vi "DEMO.vi"() -> ()   [LabVIEW 2013]
uses:
  Facade.lvclass/Facade.lvclass
  CDPlayer.lvclass/CDPlayer.lvclass
  Tuner.lvclass/Tuner.lvclass
  DVDPlayer.lvclass/DVDPlayer.lvclass
  Projector.lvclass/Projector.lvclass
  Amplifer.lvclass/Amplifer.lvclass
  RoomLight.lvclass/RoomLight.lvclass
panel:
  out "看電影的操作程序...":string
  # "表象模式簡例"
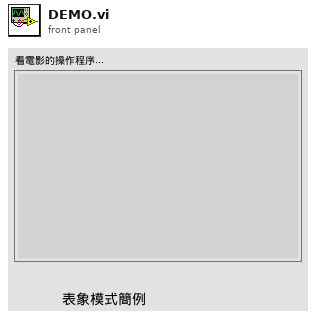
[diagram p1: front panel]
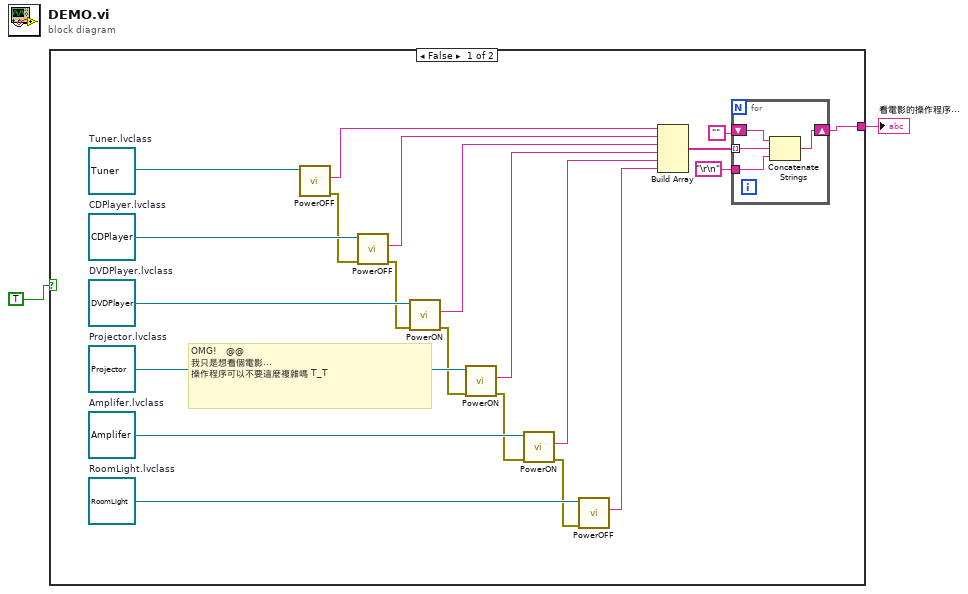
[diagram p0: block diagram]
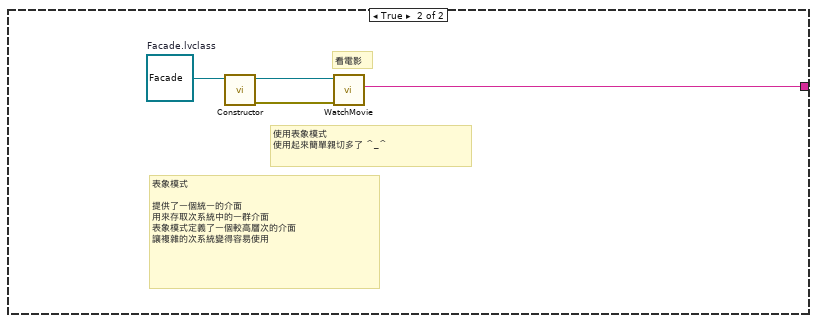
[diagram p2: hidden frame]
diagram:
  n1 = case shown="False" TRUE ("Boolean") {
    tunnel: [w23 w28] -> w2
    frame False {
      w17 = refnum<class "RoomLight.lvclass"> refnum  # RoomLight.lvclass
      w18 = refnum<class "Amplifer.lvclass"> refnum  # Amplifer.lvclass
      w19 = refnum<class "Projector.lvclass"> refnum  # Projector.lvclass
      w20 = refnum<class "DVDPlayer.lvclass"> refnum  # DVDPlayer.lvclass
      w22 = refnum<class "Tuner.lvclass"> refnum  # Tuner.lvclass
      w21 = refnum<class "CDPlayer.lvclass"> refnum  # CDPlayer.lvclass
      # "OMG!   @@\n我只是想看個電影...\n操作程序可以不要這麼複雜嗎 T_T"
      n2 = call-dynamic "PowerOFF.vi"("Tuner in"=w22) -> ("error out"=w16:errorcluster, "Message"=w8:string)  [unwired: 8 in, 1 out]
      n3 = call-dynamic "PowerOFF.vi"("error in (no error)"=w16, "CDPlayer in"=w21) -> ("error out"=w15:errorcluster, "Message"=w7:string)  [unwired: 7 in, 1 out]
      n4 = call-dynamic "PowerON.vi"("error in (no error)"=w15, "DVDPlayer in"=w20) -> ("error out"=w14:errorcluster, "Message"=w6:string)  [unwired: 7 in, 1 out]
      n5 = call-dynamic "PowerON.vi"("error in (no error)"=w14, "Projector in"=w19) -> ("error out"=w13:errorcluster, "Message"=w5:string)  [unwired: 7 in, 1 out]
      n6 = call-dynamic "PowerON.vi"("error in (no error)"=w13, "Amplifer in"=w18) -> ("error out"=w12:errorcluster, "Message"=w4:string)  [unwired: 7 in, 1 out]
      n7 = call-dynamic "PowerOFF.vi"("error in (no error)"=w12, "RoomLight in"=w17) -> ("Message"=w3:string)  [unwired: 7 in, 2 out]
      n8 = Build Array(w8, w7, w6, w5, w4, w3) -> (w11:string[])
      n9 = for {
        tunnel: w11 -> [w24] mode=indexing
        tunnel: "\r\n" -> [w27]
        shift-right: [w25] -> w23
        shift-left: "" -> [w26]
        n10 = Concatenate Strings(w26, w24, w27) -> (w25:string)
      }
    }
    frame True {
      w31 = refnum<class "Facade.lvclass"> refnum  # Facade.lvclass
      # "看電影"
      # "表象模式\n\n提供了一個統一的介面\n用來存取次系統中的一群介面\n表象模式定義了一個較高層次的介面\n讓複雜的次系統變得容易使用"
      # "使用表象模式\n使用起來簡單親切多了 ^_^"
      n11 = call-dynamic "Constructor.vi"("Facade in"=w31) -> ("error out"=w29:errorcluster, "Facade out"=w30:refnum<class "Facade.lvclass">)  [unwired: 9 in]
      n12 = call-dynamic "WatchMovie.vi"("error in (no error)"=w29, "Facade in"=w30) -> ("ProcessMessage"=w28:string)  [unwired: 7 in, 2 out]
    }
  }
  "看電影的操作程序..." <- w2
